vi "mxwScript_API_XMLConnectToInterleaveDecimateArray.vi"(5 "connectToLocation":T1, 7 "spacePerWire":u32=7, 8 "error in (no error)":errorcluster, 9 "makeSpace?":bool=TRUE, 10 "direction":T2="sink", 11 "terminalName in":string) -> (0 "error out":errorcluster, 3 "terminalName out":string)   [LabVIEW 2020]
doc: "Create encoded \"connectorPaneName\" for dynamically adding to a cluster connected to a specific connector pane terminal. The cluster is created if it does not exist using <B>clusterName</B>. If the cluster already exists, <B>clusterName</B> is ignored."
uses:
  codeGenAPISupport.llb/cgAPI_mxwScript_Wire_TerminalDirection.ctl
  codeGenAPISupport.llb/cgAPI_mxwScript_Wire_GrowableNodeConnectToLocation.ctl
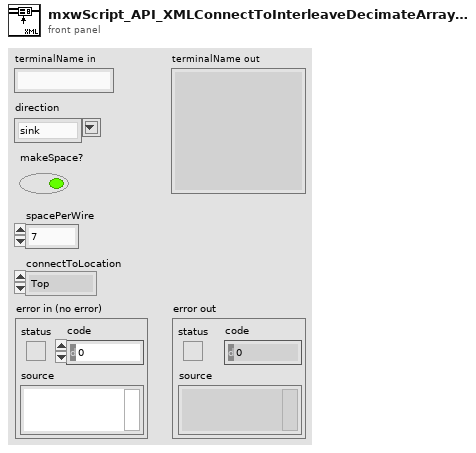
[diagram p1: front panel]
types:
  T1 = typedef "cgAPI_mxwScript_Wire_GrowableNodeConnectToLocation.ctl" = enum16{"Top", "Terminal0"}
  T2 = typedef "cgAPI_mxwScript_Wire_TerminalDirection.ctl" = string
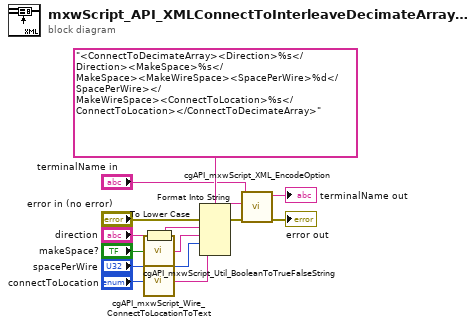
[diagram p0: block diagram]
diagram:
  n1 = To Lower Case(string="direction") -> (all lower case string=w5:T2)
  n2 = call "cgAPI_mxwScript_Util_BooleanToTrueFalseString.vi"("boolean"="makeSpace?") -> ("TRUE/FALSE text"=w7:string)  [unwired: 4 out]
  n3 = call "cgAPI_mxwScript_Wire_ConnectToLocationToText.vi"("connectToLocation"="connectToLocation") -> ("resulting string"=w1:string)  [unwired: 4 out]
  n4 = Format Into String(format string="<ConnectToDecimateArray><Direction>%s</Direction><MakeSpace>%s</MakeSpace><MakeWireSpace><SpacePerWire>%d</SpacePerWire></MakeWireSpace><ConnectToLocation>%s</ConnectToLocation></ConnectToDecimateArray>" ("control name"), error in="error in (no error)", w5, w7, "spacePerWire", w1) -> (resulting string=w10:string, error out=w12:errorcluster)  [unwired: 1 in]
  n5 = call "cgAPI_mxwScript_XML_EncodeOption.vi"("error in (no error)"=w12, "otherXML"=w10, "normalTextString"="terminalName in") -> ("error out"=→"error out":errorcluster, "encodedString"=→"terminalName out":string)  [unwired: 7 out]
